vi "Area triangulo.vi"() -> ()   [LabVIEW 2019]
panel:
  out "Numeric 3":dbl
  in  "Numeric 2":dbl
  in  "Numeric":dbl
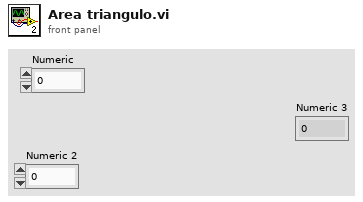
[diagram p1: front panel]
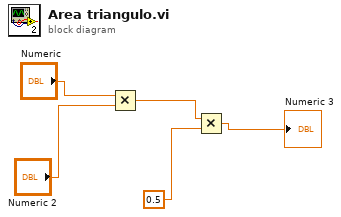
[diagram p0: block diagram]
diagram:
  n1 = Multiply(x="Numeric", y="Numeric 2") -> (x*y=w4:dbl)
  n2 = Multiply(x=w4, y=0.5) -> (x*y=→"Numeric 3":dbl)
